vi "Control Panel.vi"(8 "error in (no error)":errorcluster, 11 "Fake Pulse Generator in":refnum<class "Pulse Generator.lvclass">) -> (0 "error out":errorcluster, 3 "Fake Pulse Generator out":refnum<class "Pulse Generator.lvclass">)   [LabVIEW 2009, in "Pulse Generator.lvclass"]
uses:
  Pulse Generator.lvclass
  Utility Classes/Scannable/Scannable.lvclass
  Pulse Generator.lvclass/Pulse Generator.ctl
panel:
  in  "Width/Duty\nUP/DOWN Ch2":bool
  in  "Width/Duty\nUP/DOWN Ch1":bool
  in  "Clear Error":bool
  out "Ready when \nblinking":bool
  in  "Copy actual to set":bool
  out "Pulse Mode":enum16{"Pulses", "Pattern"}(ring)
  out "Arming (Trigger) Source":T1(ring)
  in  "Populate fields with member data":bool
  out "Strobe Pattern":string
  in  "Strobe Pattern Set":string
  out "StrobeDataBuffer":digitalwaveform(graph)
  in  "Enable/disable":bool
  in  "Modes (changes immediately)":T2(radio)
  in  "BitPeriodSet":dbl[unit]
  out "BitPeriod":dbl[unit]
  out "Ch2Pattern":string
  in  "Ch2Pattern Set":string
  out "Ch1Pattern":string
  in  "Set Patterns":bool
  in  "Ch1Pattern Set":string
  in  "Ch2Duty (%) Set":dbl=10.0
  in  "Ch1Duty (%) Set":dbl=10.0
  in  "Ch1Delay Set":dbl[unit]
  in  "Ch2Delay Set":dbl[unit]
  in  "stop":bool
  out "Ch1DataBuffer":digitalwaveform(graph)
  out "Ch2DataBuffer":digitalwaveform(graph)
  in  "Ch2 Sync":bool
  in  "Ch1 Sync":bool
  in  "Ch2 Toggle":bool
  in  "Ch1 NOT Toggle":bool
  in  "Ch1 Toggle":bool
  in  "Ch2 NOT Toggle":bool
  in  "OverallPeriodSet":dbl[unit]
  in  "Ch2WidthSet":dbl[unit]=1e-09
  in  "Ch1WidthSet":dbl[unit]=1e-09
  in  "Ch2LowSet":dbl[unit]
  in  "Ch2HighSet":dbl[unit]
  in  "Ch1LowSet":dbl[unit]
  in  "Ch1HighSet":dbl[unit]
  in  "OverallFreqSet":dbl[unit]
  in  "Read to Control":bool
  in  "Set":bool
  out "Ch2Duty (%)":dbl
  out "Ch1Duty (%)":dbl
  out "Ch1Delay":dbl[unit]
  out "Ch2Delay":dbl[unit]
  out "Ch1Low":dbl[unit]
  out "Ch1High":dbl[unit]
  out "Ch2Width":dbl[unit]
  out "Ch1Width":dbl[unit]
  out "OverallPeriod":dbl[unit]
  out "Ch2Low":dbl[unit]
  out "Ch2High":dbl[unit]
  in  "Read":bool
  out "OverallFreq":dbl[unit]
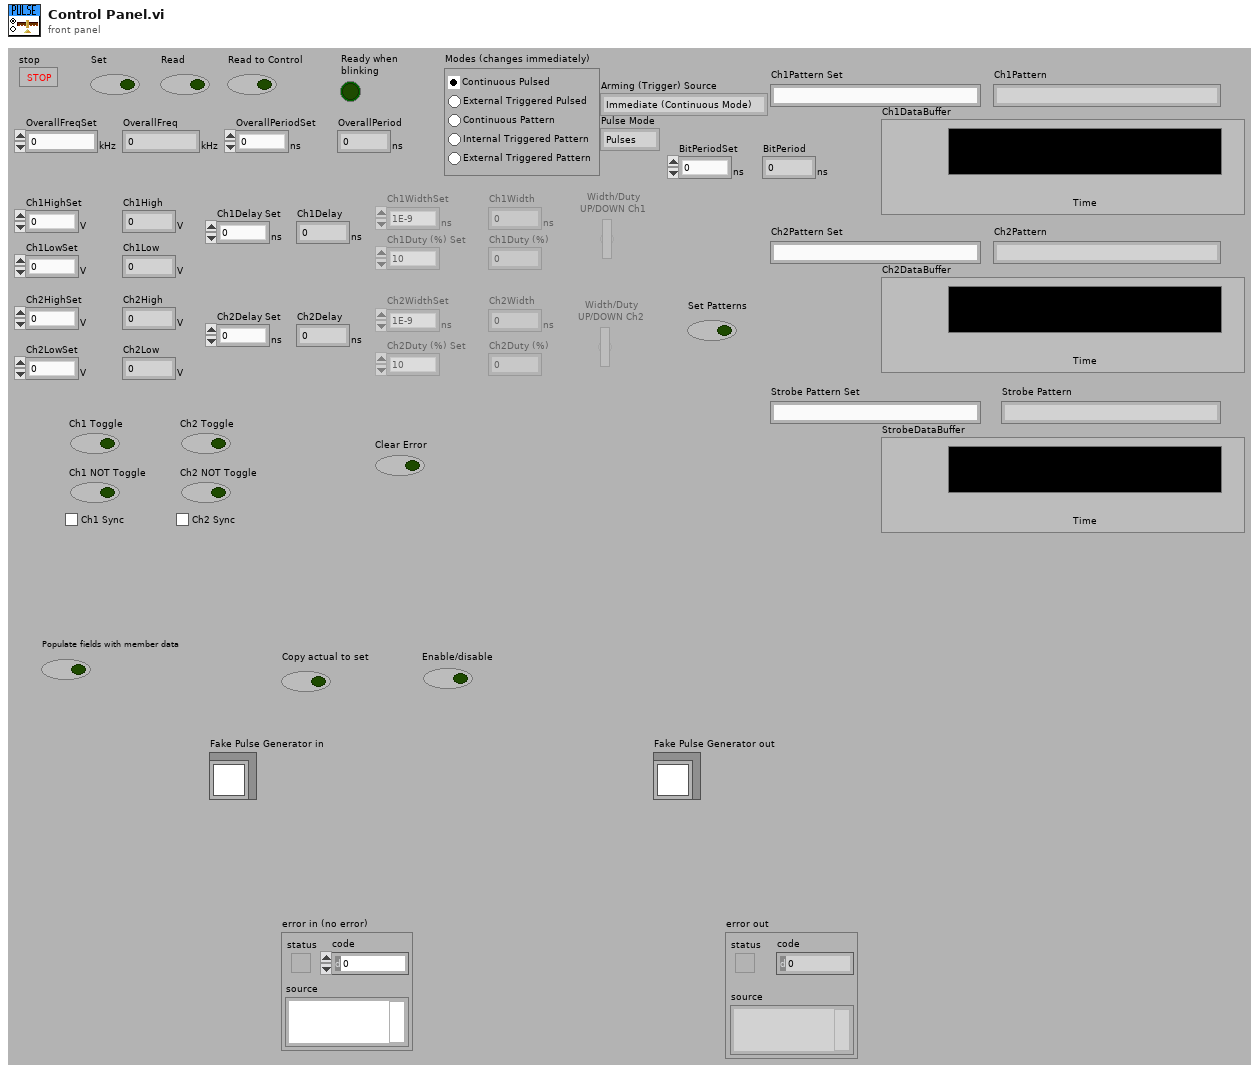
[diagram p1: front panel]
types:
  T1 = enum16{"Immediate (Continuous Mode)", "Internal PLL", "External", "Manual"}
  T2 = enum32{"Continuous Pulsed", "Continuous Pattern", "Internal Triggered Pattern", "External Triggered Pulsed", "External Triggered Pattern", "Other"}
  T3 = enum16{"Internal Oscillator", "Internal PLL", "External Clock "}
  T4 = enum16{"Internal Oscillator", "Internal PLL", "Clock Input"}
  T5 = enum16{"Channel All ", "Channel 1", "Channel 2", "Channel 3", "Channels Combined"}
  T6 = cluster{"1 High":dbl[unit], "1 Low":dbl[unit], "2 High":dbl[unit], "2 Low":dbl[unit]}
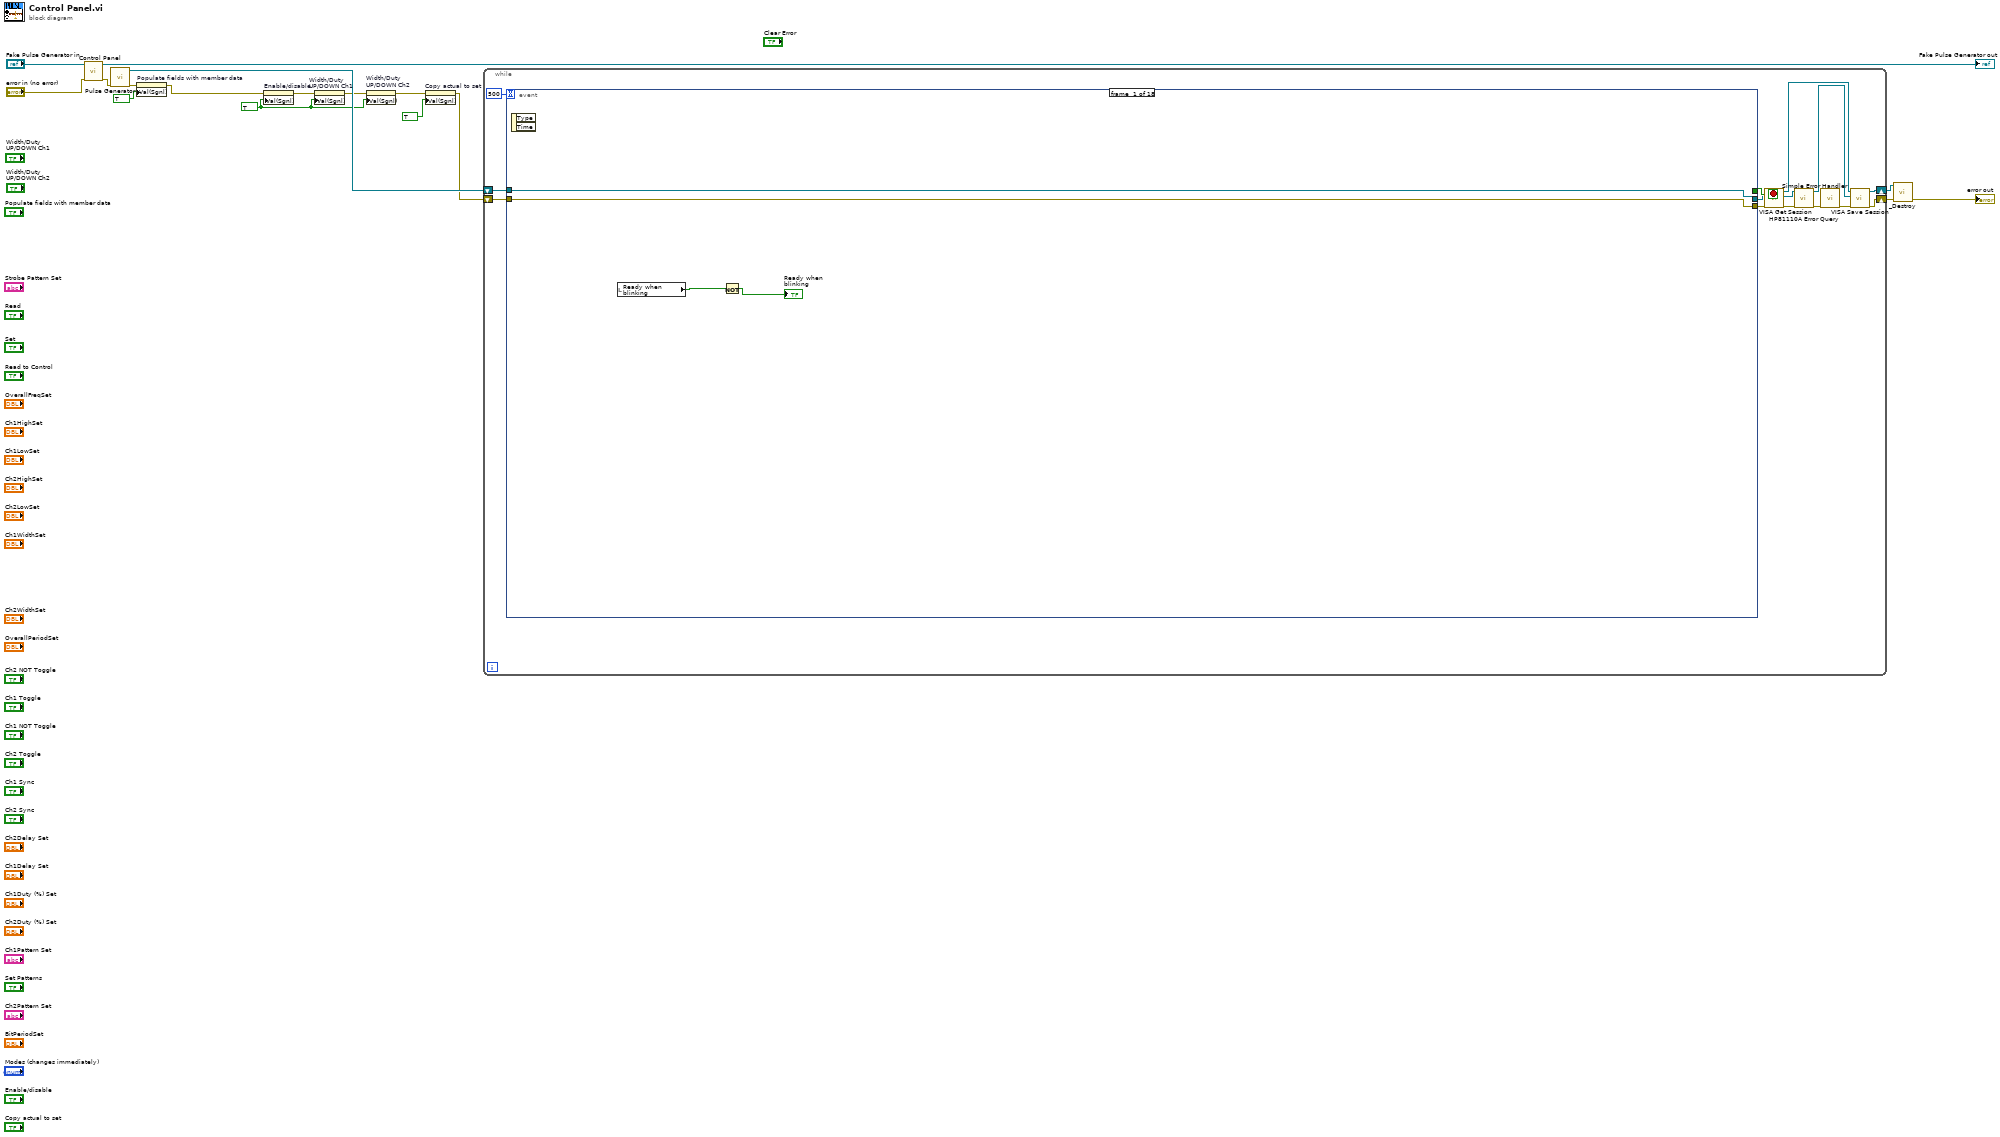
[diagram p0: block diagram]
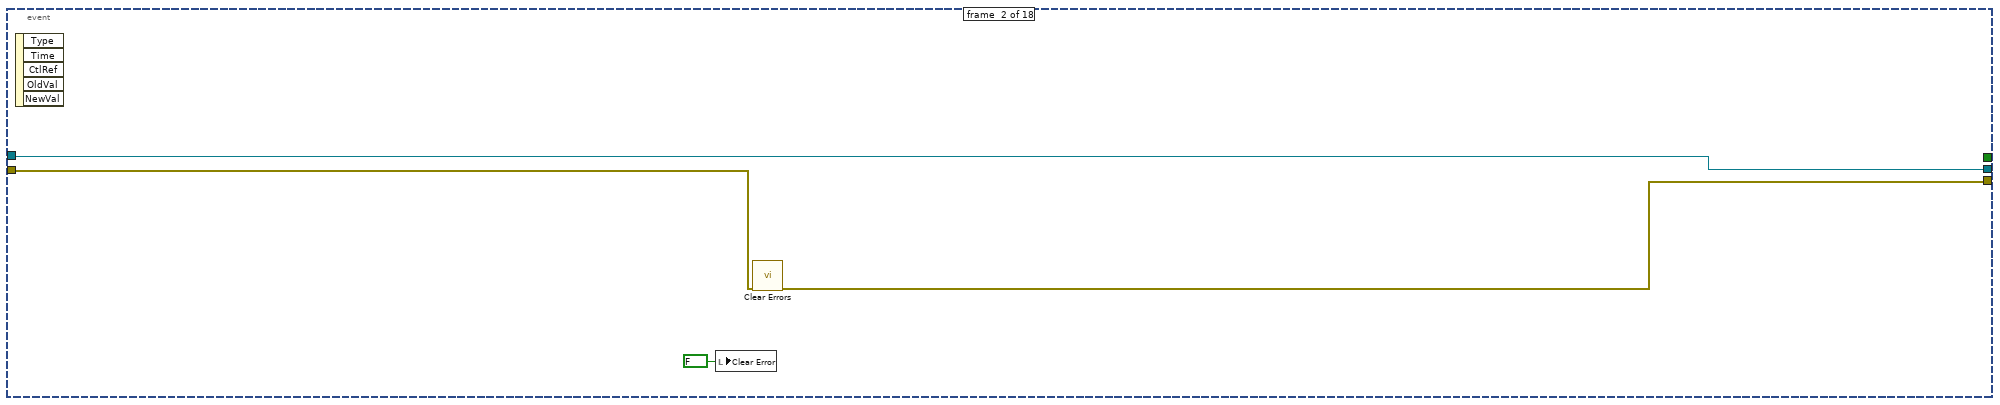
[diagram p2: hidden frame]
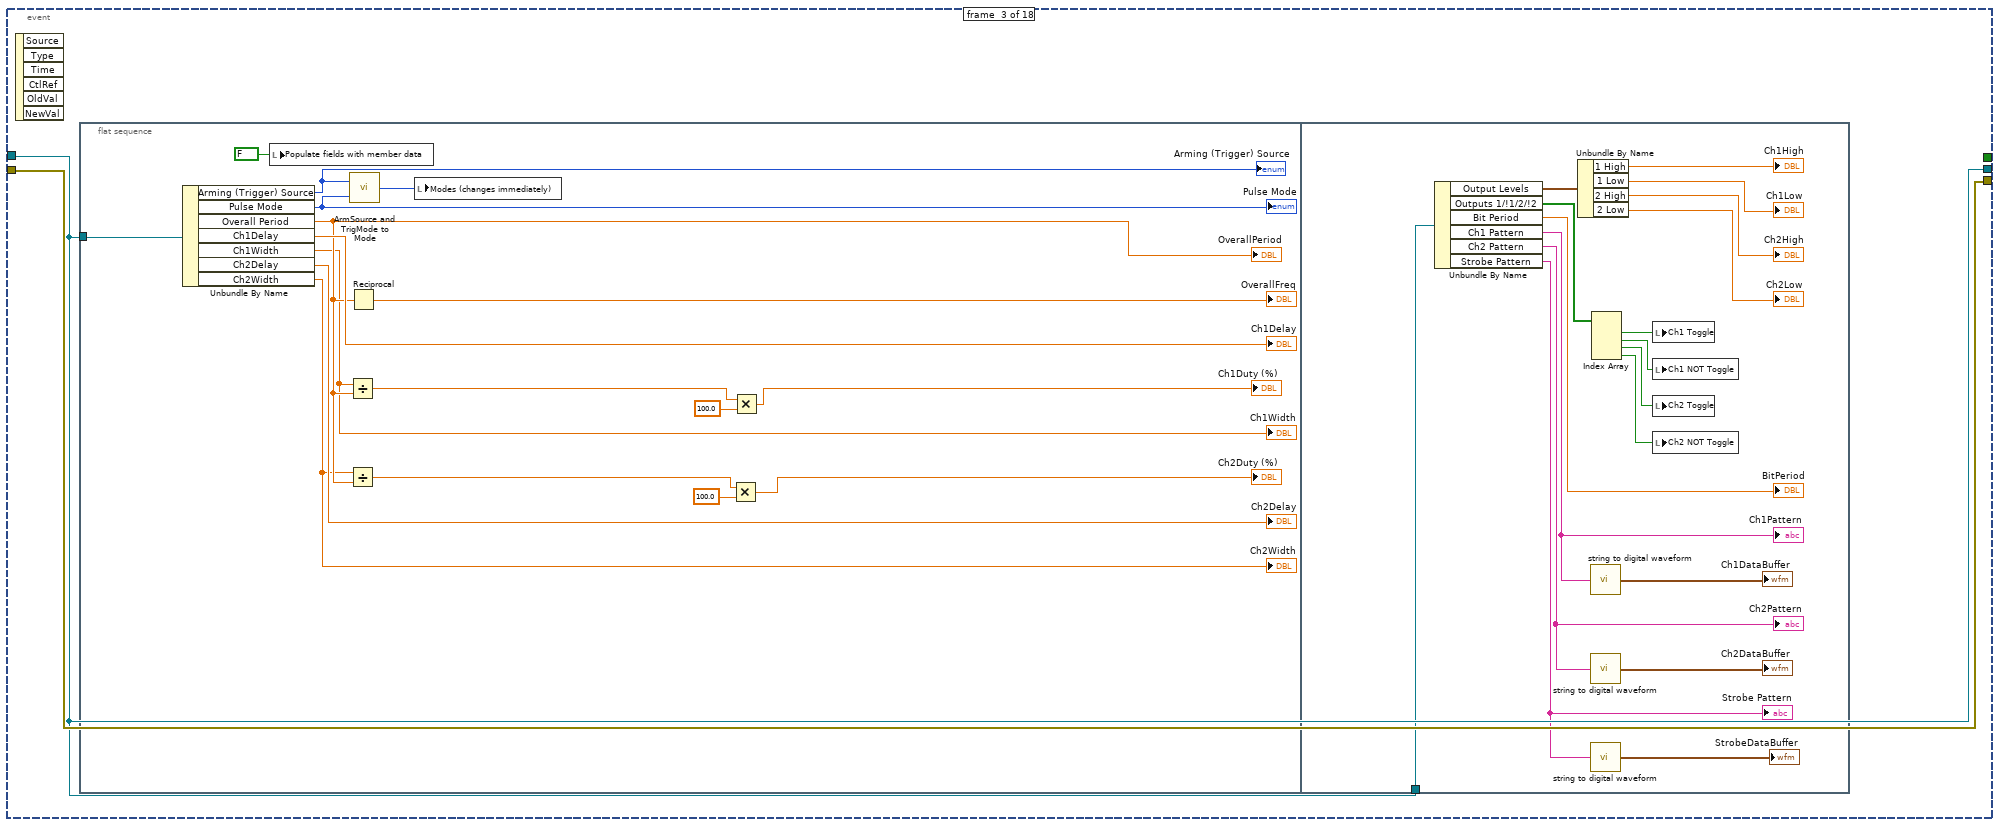
[diagram p3: hidden frame]
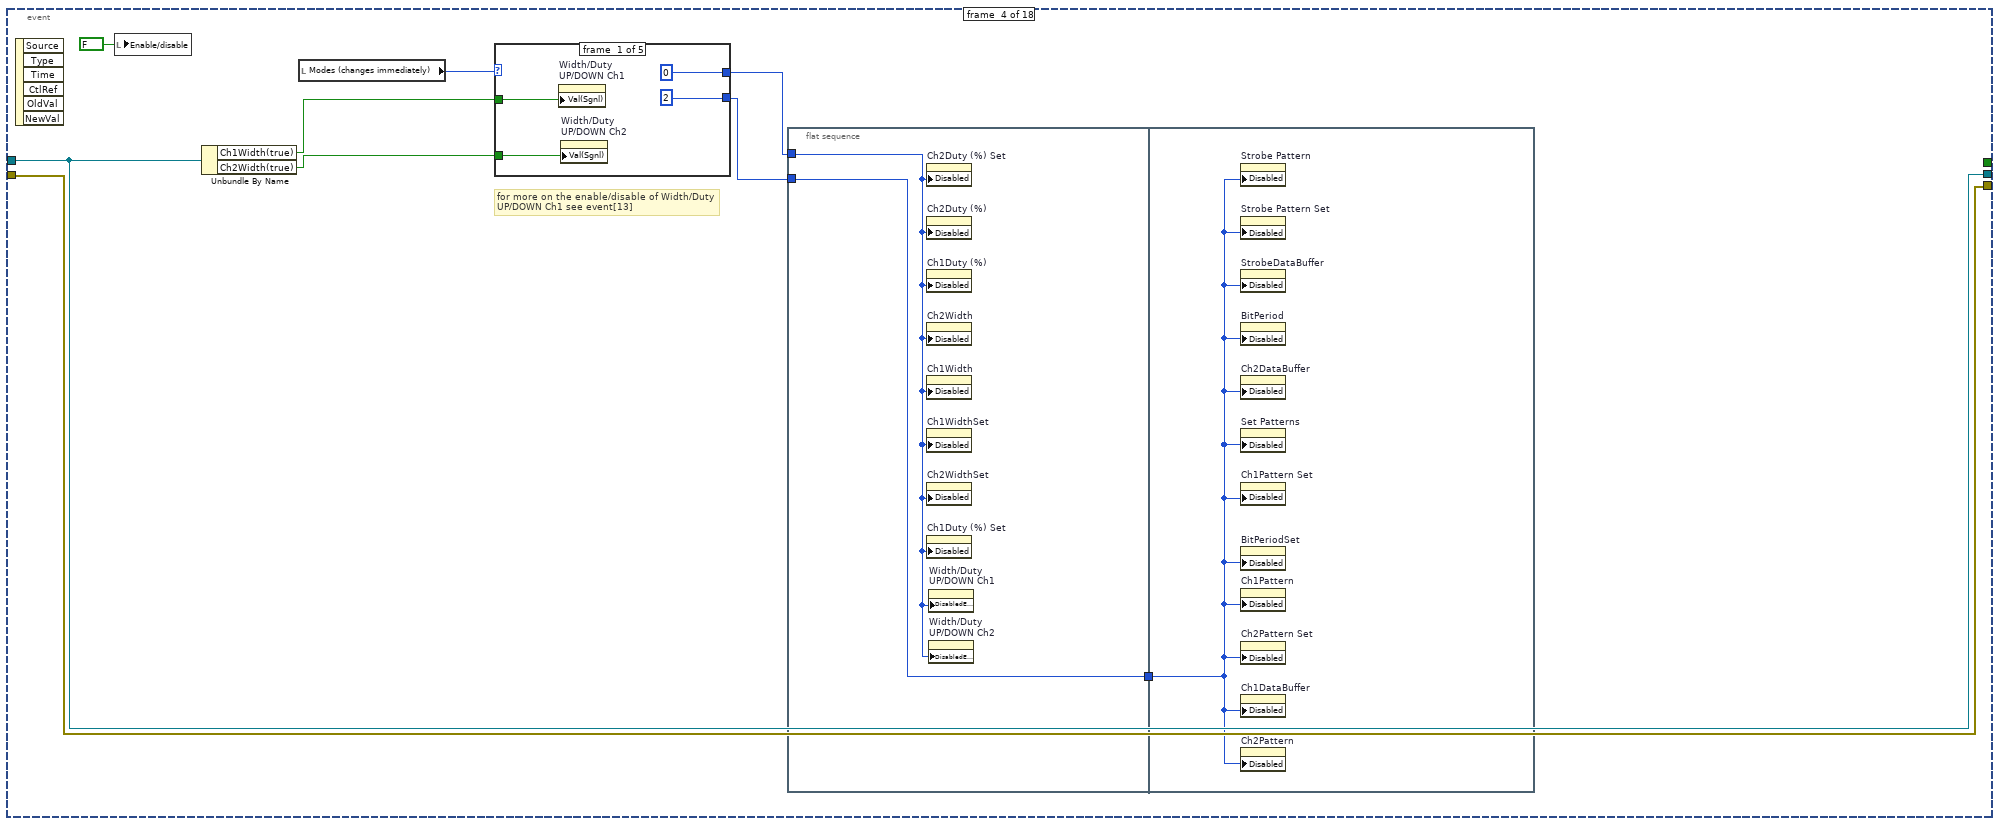
[diagram p4: hidden frame]
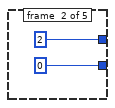
[diagram p5: hidden frame]
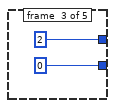
[diagram p6: hidden frame]
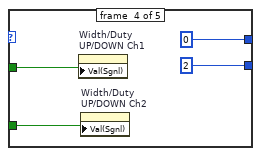
[diagram p7: hidden frame]
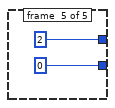
[diagram p8: hidden frame]
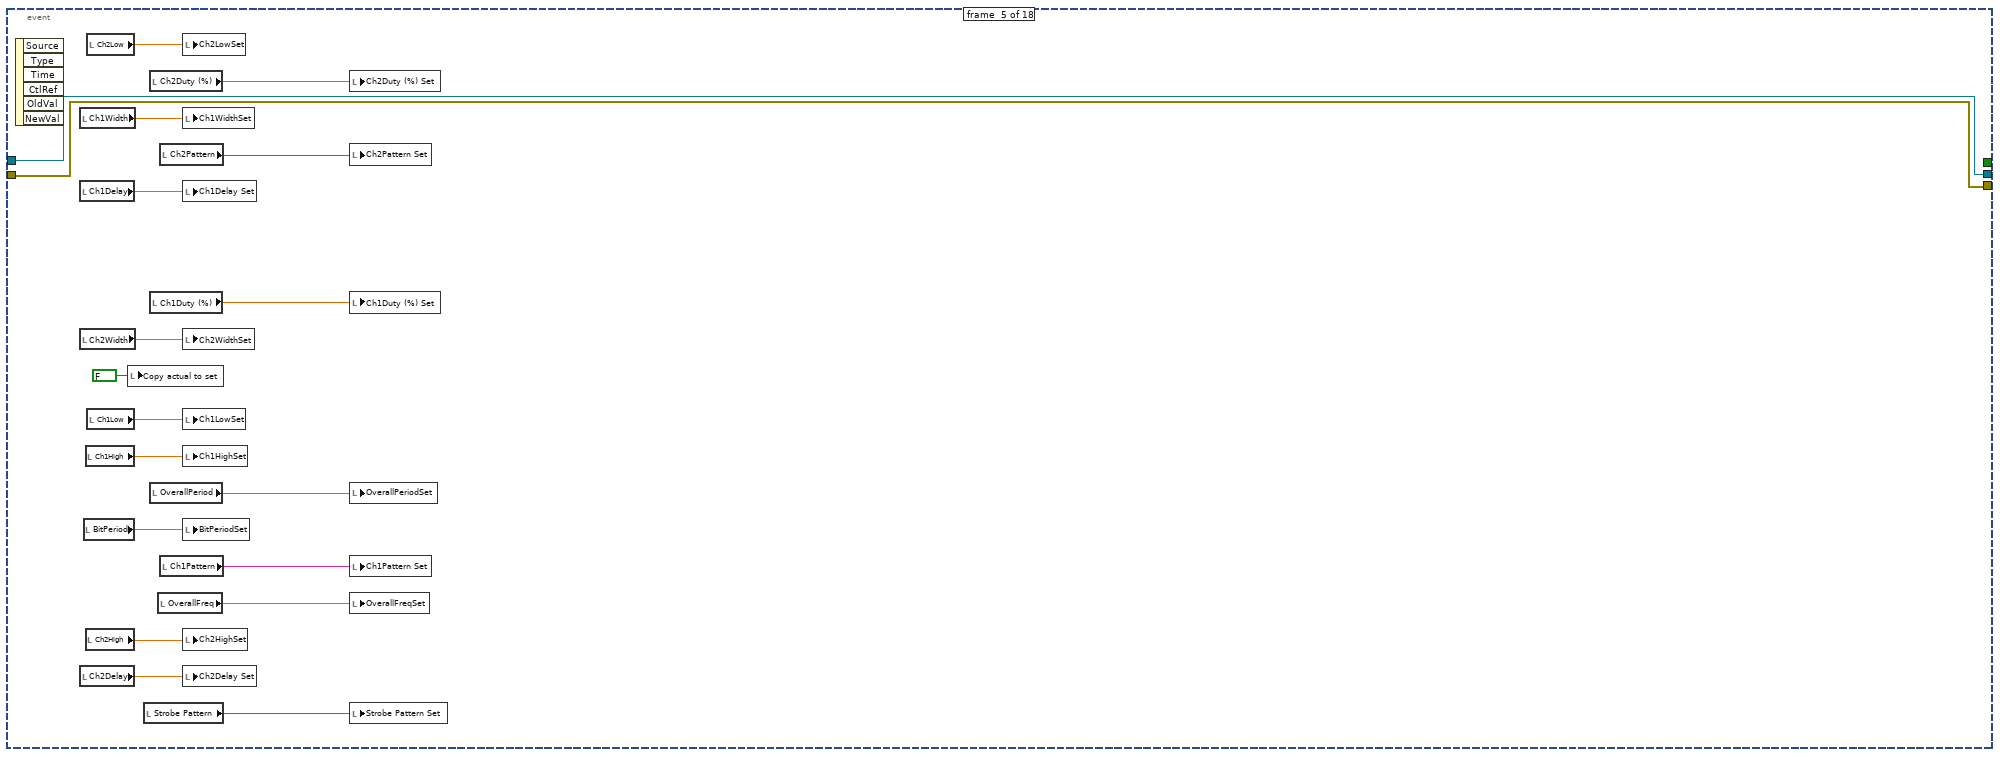
[diagram p9: hidden frame]
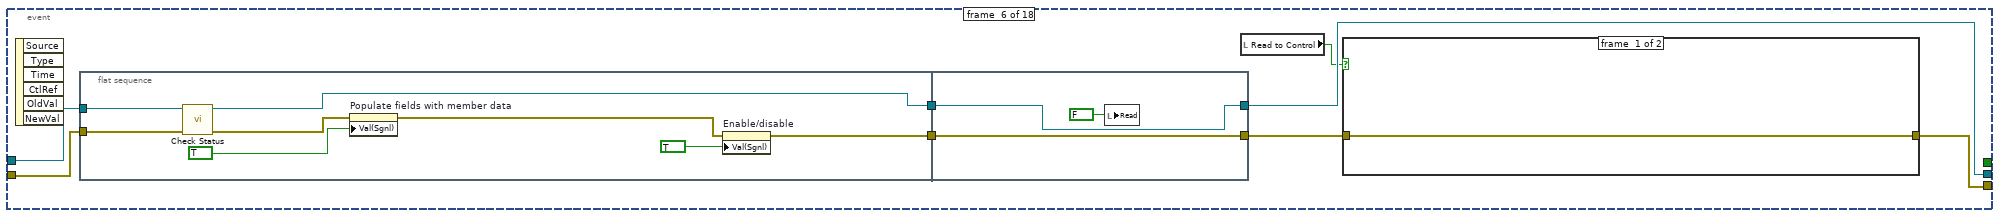
[diagram p10: hidden frame]
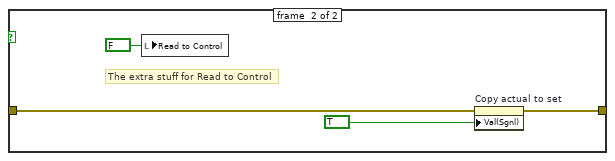
[diagram p11: hidden frame]
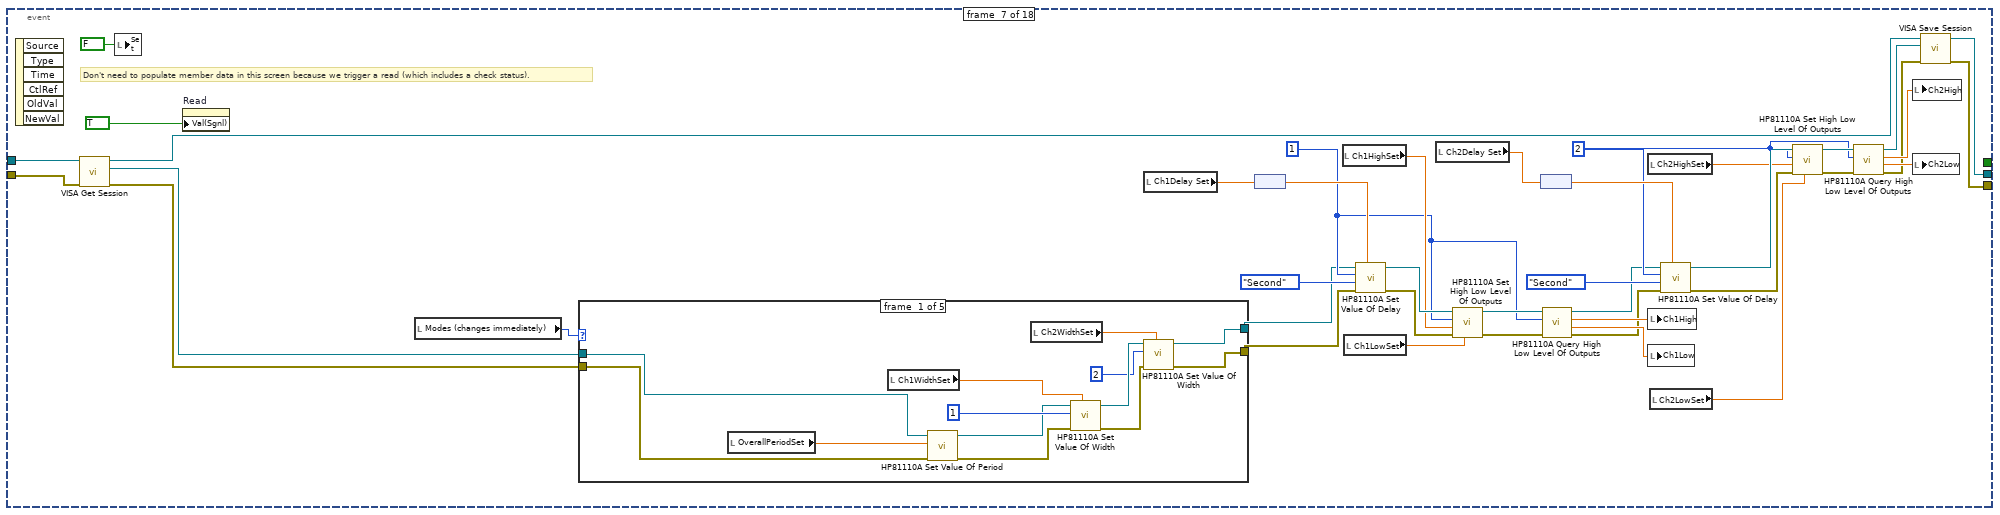
[diagram p12: hidden frame]
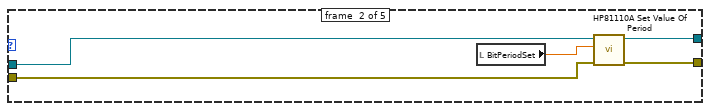
[diagram p13: hidden frame]
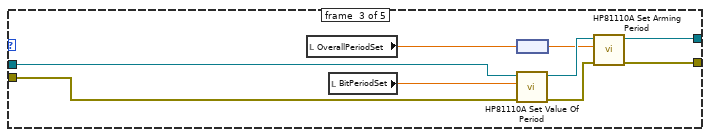
[diagram p14: hidden frame]
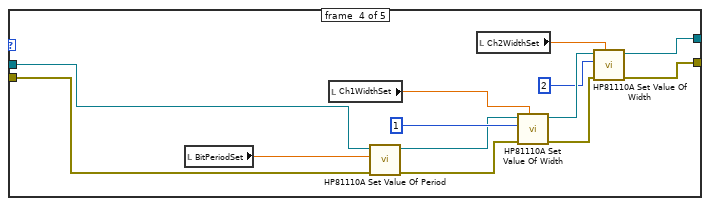
[diagram p15: hidden frame]
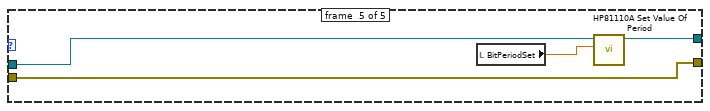
[diagram p16: hidden frame]
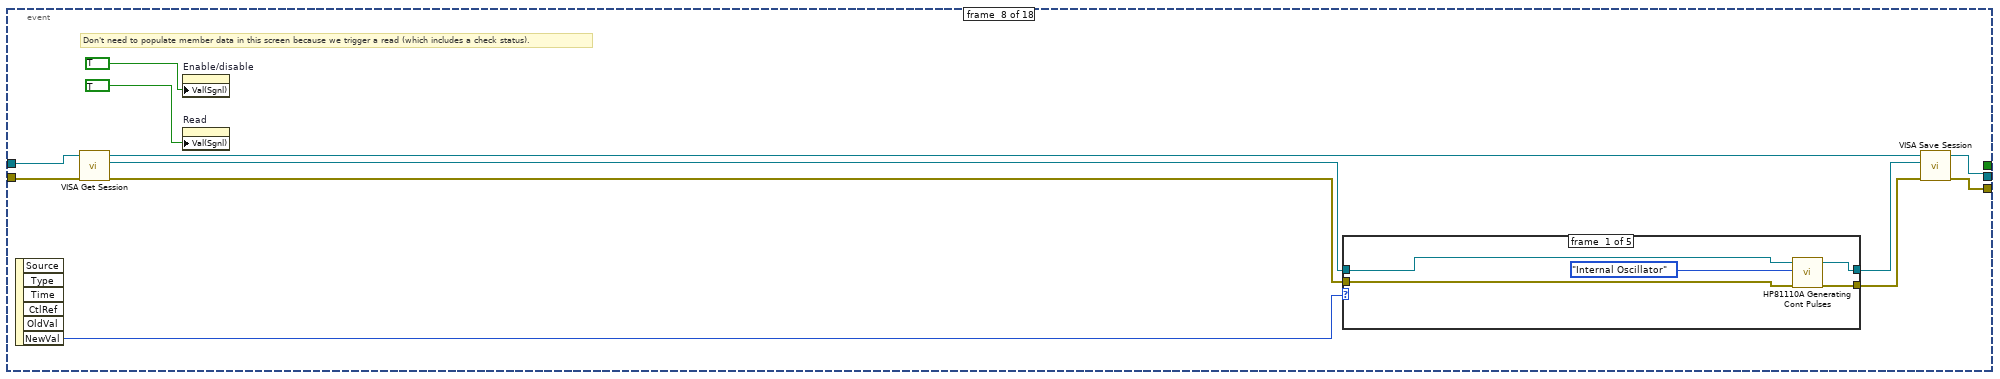
[diagram p17: hidden frame]
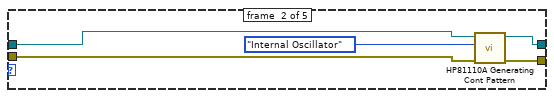
[diagram p18: hidden frame]
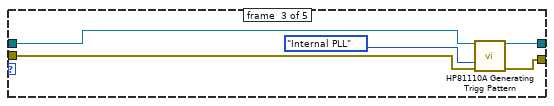
[diagram p19: hidden frame]
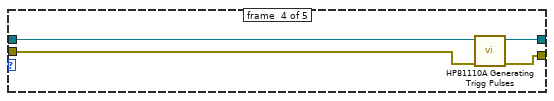
[diagram p20: hidden frame]
diagram:
  w1 = TRUE ("Value (Signaling)")
  n1 = call-parent "Control Panel.vi"("error in (no error)"="error in (no error)", "Instrument in"="Fake Pulse Generator in") -> ("error out"=w8:errorcluster, "Instrument out"=→"Fake Pulse Generator out":refnum<class "Pulse Generator.lvclass">)  [unwired: 8 out]
  n2 = call "Pulse Generator.vi"("error in (no error)"=w8) -> ("error out"=w9:errorcluster, "Pulse Generator out"=w14:refnum<class "Pulse Generator.lvclass">)  [unwired: 9 out]
  n3 = property on="Populate fields with member data" class="Bool (strict)"(error in=w9, "Val(Sgnl)"=TRUE ("Value (Signaling)")) -> (error out=w6:errorcluster)  [unwired: 1 in, 1 out]
  n4 = property on="Enable/disable" class="Bool (strict)"(error in=w6, "Val(Sgnl)"=w1) -> (error out=w4:errorcluster)  [unwired: 1 in, 1 out]
  n5 = property on="Width/Duty\nUP/DOWN Ch1" class="Bool (strict)"(error in=w4, "Val(Sgnl)"=w1) -> (error out=w2:errorcluster)  [unwired: 1 in, 1 out]
  n6 = property on="Width/Duty\nUP/DOWN Ch2" class="Bool (strict)"(error in=w2, "Val(Sgnl)"=w1) -> (error out=w3:errorcluster)  [unwired: 1 in, 1 out]
  n7 = property on="Copy actual to set" class="Bool (strict)"(error in=w3, "Val(Sgnl)"=TRUE ("Value (Signaling)")) -> (error out=w5:errorcluster)  [unwired: 1 in, 1 out]
  n8 = while {
    shift-right: [w24] -> w13
    shift-left: w14 -> [w29]
    shift-right: [w19] -> w12
    shift-left: w5 -> [w28]
    stop <- w31 stop-if-true
    n9 = event shown="[2] \"Populate fields with member data\": Value Change" {
      selector: _ -> [_ _ _ _ _ _ _ _ _ _ _ _ _ _ _ _ _ _]
      dyn-events: _ -> [_ _ _ _ _ _ _ _ _ _ _ _ _ _ _ _ _ _]
      timeout: 500 -> [_ _ _ _ _ _ _ _ _ _ _ _ _ _ _ _ _ _]
      tunnel: [_ _ _ _ _ _ _ _ _ _ _ _ "stop" _ _ _ _ _] -> w31
      tunnel: w28 -> [w34 w39 w41 w84 w104 w129 w152 w236 w274 w302 w312 w335 w348 w368 w370 w380 w390 w396]
      tunnel: [w34 w37 w41 w84 w104 w125 w147 w232 w268 w300 w312 w335 w348 w368 w370 w380 w390 w396] -> w22
      tunnel: w29 -> [w35 w38 w40 w79 w105 w128 w154 w238 w275 w303 w313 w336 w347 w355 w369 w379 w389 w397]
      tunnel: [w35 w38 w40 w79 w105 w127 w149 w233 w270 w291 w313 w336 w347 w354 w369 w379 w389 w397] -> w23
      event #0 {
        n10 = event-data() -> ()  [unwired: 3 out]
        n11 = local read "Ready when \nblinking"() -> (w33:bool)
        n12 = Not(x=w33) -> (.not. x?=→"Ready when \nblinking":bool)
      }
      event #1 {
        n13 = event-data() -> ()  [unwired: 6 out]
        n14 = local write "Clear Error"(FALSE ("Clear Error")) -> ()
        n15 = call <vilib>:"Clear Errors.vi"("error in (no error)"=w39) -> ("error out"=w37:errorcluster)  [unwired: 6 in]
      }
      event #2 {
        n16 = event-data() -> ()  [unwired: 7 out]
        n17 = flat-sequence {
          tunnel: w40 -> [w48]
          tunnel: w40 -> [w59]
          frame #0 {
            n18 = Unbundle By Name(w48) -> ("Arming (Trigger) Source"=w51:u16, "Pulse Mode"=w50:u16, "Overall Period"=w54:dbl[unit], "Ch1Delay"=→"Ch1Delay":dbl[unit], "Ch1Width"=w53:dbl[unit], "Ch2Delay"=→"Ch2Delay":dbl[unit], "Ch2Width"=w52:dbl[unit])
            "OverallPeriod" <- w54
            "Ch1Width" <- w53
            "Ch2Width" <- w52
            "Arming (Trigger) Source" <- w51
            "Pulse Mode" <- w50
            n19 = local write "Populate fields with member data"(FALSE ("Populate fields with member data")) -> ()
            n20 = Divide(x=w53, y=w54) -> (x/y=w45:dbl)
            n21 = Divide(x=w52, y=w54) -> (x/y=w43:dbl)
            n22 = Reciprocal(x=w54) -> (1/x=→"OverallFreq":dbl[unit])
            n23 = call "ArmSource and TrigMode to Mode.vi"("Pulse Mode"=w50, "Arming (Trigger) Source (0:Internal PLL)"=w51) -> ("Modes (changes immediately)"=w49:T2)
            n24 = local write "Modes (changes immediately)"(w49) -> ()
            n25 = Multiply(x=w43, y=100.0) -> (x*y=→"Ch2Duty (%)":dbl)
            n26 = Multiply(x=w45, y=100.0) -> (x*y=→"Ch1Duty (%)":dbl)
          }
          frame #1 {
            n27 = Unbundle By Name(w59) -> ("Output Levels"=w71:T6, "Outputs 1/!1/2/!2"=w72:bool[], "Bit Period"=→"BitPeriod":dbl[unit], "Ch1 Pattern"=w74:string, "Ch2 Pattern"=w75:string, "Strobe Pattern"=w76:string)
            "Ch1Pattern" <- w74
            "Ch2Pattern" <- w75
            "Strobe Pattern" <- w76
            n28 = Unbundle By Name(w71) -> ("1 High"=→"Ch1High":dbl[unit], "1 Low"=→"Ch1Low":dbl[unit], "2 High"=→"Ch2High":dbl[unit], "2 Low"=→"Ch2Low":dbl[unit])
            n29 = call "string to digital waveform.vi"("String"=w74) -> ("digital waveform"=→"Ch1DataBuffer":digitalwaveform)
            n30 = call "string to digital waveform.vi"("String"=w75) -> ("digital waveform"=→"Ch2DataBuffer":digitalwaveform)
            n31 = call "string to digital waveform.vi"("String"=w76) -> ("digital waveform"=→"StrobeDataBuffer":digitalwaveform)
            n32 = Index Array(array=w72) -> (element #1=w67:bool, element #2=w68:bool, element #3=w69:bool, element #4=w70:bool)  [unwired: 4 in]
            n33 = local write "Ch1 Toggle"(w67) -> ()
            n34 = local write "Ch1 NOT Toggle"(w68) -> ()
            n35 = local write "Ch2 Toggle"(w69) -> ()
            n36 = local write "Ch2 NOT Toggle"(w70) -> ()
          }
        }
      }
      event #3 {
        # "for more on the enable/disable of Width/Duty\nUP/DOWN Ch1 see event[13]"
        n37 = event-data() -> ()  [unwired: 7 out]
        n38 = local write "Enable/disable"(FALSE ("Enable/disable")) -> ()
        n39 = Unbundle By Name(w79) -> ("Ch1Width(true)"=w77:bool, "Ch2Width(true)"=w78:bool)
        n40 = local read "Modes (changes immediately)"() -> (w82:T2)
        n41 = case shown="\"External Triggered Pulsed\"" w82 {
          tunnel: [2 0 0 2 0] -> w80
          tunnel: [0 2 2 0 2] -> w81
          tunnel: w78 -> [w87 _ _ w94 _]
          tunnel: w77 -> [w86 _ _ w95 _]
          frame #0 {
            n42 = property on="Width/Duty\nUP/DOWN Ch1" class="Bool (strict)"("Val(Sgnl)"=w86) -> ()  [unwired: 2 in, 2 out]
            n43 = property on="Width/Duty\nUP/DOWN Ch2" class="Bool (strict)"("Val(Sgnl)"=w87) -> ()  [unwired: 2 in, 2 out]
          }
          frame #1 {
          }
          frame #2 {
          }
          frame #3 {
            n44 = property on="Width/Duty\nUP/DOWN Ch1" class="Bool (strict)"("Val(Sgnl)"=w95) -> ()  [unwired: 2 in, 2 out]
            n45 = property on="Width/Duty\nUP/DOWN Ch2" class="Bool (strict)"("Val(Sgnl)"=w94) -> ()  [unwired: 2 in, 2 out]
          }
          frame #4 {
          }
        }
        n46 = flat-sequence {
          tunnel: [w101] -> w83
          tunnel: w81 -> [w100]
          tunnel: w80 -> [w101]
          tunnel: w83 -> [w102]
          frame #0 {
            n47 = property on="Ch2Duty (%) Set" class="DigNum (strict)"("Disabled"=w100) -> ()  [unwired: 2 in, 2 out]
            n48 = property on="Ch2Duty (%)" class="DigNum (strict)"("Disabled"=w100) -> ()  [unwired: 2 in, 2 out]
            n49 = property on="Ch1Duty (%)" class="DigNum (strict)"("Disabled"=w100) -> ()  [unwired: 2 in, 2 out]
            n50 = property on="Ch2Width" class="DigNum (strict)"("Disabled"=w100) -> ()  [unwired: 2 in, 2 out]
            n51 = property on="Ch1Width" class="DigNum (strict)"("Disabled"=w100) -> ()  [unwired: 2 in, 2 out]
            n52 = property on="Ch1WidthSet" class="DigNum (strict)"("Disabled"=w100) -> ()  [unwired: 2 in, 2 out]
            n53 = property on="Ch2WidthSet" class="DigNum (strict)"("Disabled"=w100) -> ()  [unwired: 2 in, 2 out]
            n54 = property on="Ch1Duty (%) Set" class="DigNum (strict)"("Disabled"=w100) -> ()  [unwired: 2 in, 2 out]
            n55 = property on="Width/Duty\nUP/DOWN Ch1" class="Bool (strict)"("DisabledEnum"=w100) -> ()  [unwired: 2 in, 2 out]
            n56 = property on="Width/Duty\nUP/DOWN Ch2" class="Bool (strict)"("DisabledEnum"=w100) -> ()  [unwired: 2 in, 2 out]
          }
          frame #1 {
            n57 = property on="Strobe Pattern" class="Str"("Disabled"=w102) -> ()  [unwired: 2 in, 2 out]
            n58 = property on="Strobe Pattern Set" class="Str"("Disabled"=w102) -> ()  [unwired: 2 in, 2 out]
            n59 = property on="StrobeDataBuffer" class="DigitalGraph (strict)"("Disabled"=w102) -> ()  [unwired: 2 in, 2 out]
            n60 = property on="BitPeriod" class="DigNum (strict)"("Disabled"=w102) -> ()  [unwired: 2 in, 2 out]
            n61 = property on="Ch2DataBuffer" class="DigitalGraph (strict)"("Disabled"=w102) -> ()  [unwired: 2 in, 2 out]
            n62 = property on="Set Patterns" class="Bool (strict)"("Disabled"=w102) -> ()  [unwired: 2 in, 2 out]
            n63 = property on="Ch1Pattern Set" class="Str"("Disabled"=w102) -> ()  [unwired: 2 in, 2 out]
            n64 = property on="BitPeriodSet" class="DigNum (strict)"("Disabled"=w102) -> ()  [unwired: 2 in, 2 out]
            n65 = property on="Ch1Pattern" class="Str"("Disabled"=w102) -> ()  [unwired: 2 in, 2 out]
            n66 = property on="Ch2Pattern Set" class="Str"("Disabled"=w102) -> ()  [unwired: 2 in, 2 out]
            n67 = property on="Ch1DataBuffer" class="DigitalGraph (strict)"("Disabled"=w102) -> ()  [unwired: 2 in, 2 out]
            n68 = property on="Ch2Pattern" class="Str"("Disabled"=w102) -> ()  [unwired: 2 in, 2 out]
          }
        }
      }
      event #4 {
        n69 = event-data() -> ()  [unwired: 7 out]
        n70 = local read "Ch1Width"() -> (w117:dbl[unit])
        n71 = local read "Ch1Delay"() -> (w115:dbl[unit])
        n72 = local read "Ch2Width"() -> (w113:dbl[unit])
        n73 = local read "Ch2Delay"() -> (w111:dbl[unit])
        n74 = local read "BitPeriod"() -> (w107:dbl[unit])
        n75 = local read "Ch1High"() -> (w119:dbl[unit])
        n76 = local read "Ch2High"() -> (w110:dbl[unit])
        n77 = local read "Ch2Low"() -> (w114:dbl[unit])
        n78 = local read "Ch1Low"() -> (w118:dbl[unit])
        n79 = local write "Copy actual to set"(FALSE ("Copy actual to set")) -> ()
        n80 = local read "Strobe Pattern"() -> (w103:string)
        n81 = local read "Ch2Duty (%)"() -> (w112:dbl)
        n82 = local read "Ch1Duty (%)"() -> (w116:dbl)
        n83 = local read "OverallPeriod"() -> (w120:dbl[unit])
        n84 = local read "OverallFreq"() -> (w121:dbl[unit])
        n85 = local read "Ch2Pattern"() -> (w108:string)
        n86 = local read "Ch1Pattern"() -> (w109:string)
        n87 = local write "Ch2LowSet"(w114) -> ()
        n88 = local write "Ch1WidthSet"(w117) -> ()
        n89 = local write "Ch1Delay Set"(w115) -> ()
        n90 = local write "Ch2WidthSet"(w113) -> ()
        n91 = local write "Ch1LowSet"(w118) -> ()
        n92 = local write "Ch1HighSet"(w119) -> ()
        n93 = local write "BitPeriodSet"(w107) -> ()
        n94 = local write "Ch2HighSet"(w110) -> ()
        n95 = local write "Ch2Delay Set"(w111) -> ()
        n96 = local write "Ch2Duty (%) Set"(w112) -> ()
        n97 = local write "Ch2Pattern Set"(w108) -> ()
        n98 = local write "Ch1Duty (%) Set"(w116) -> ()
        n99 = local write "OverallPeriodSet"(w120) -> ()
        n100 = local write "Ch1Pattern Set"(w109) -> ()
        n101 = local write "OverallFreqSet"(w121) -> ()
        n102 = local write "Strobe Pattern Set"(w103) -> ()
      }
      event #5 {
        n103 = event-data() -> ()  [unwired: 7 out]
        n104 = flat-sequence {
          tunnel: w129 -> [w137]
          tunnel: w128 -> [w136]
          tunnel: [w135] -> w123
          tunnel: [w134] -> w122
          tunnel: [w139] -> w126
          tunnel: [w140] -> w127
          tunnel: w123 -> [w140]
          tunnel: w122 -> [w139]
          frame #0 {
            n105 = call-dynamic "Check Status.vi"("error in (no error)"=w137, "Pulse Generator in"=w136) -> ("error out"=w131:errorcluster, "Pulse Generator out"=w135:refnum<class "Pulse Generator.lvclass">)  [unwired: 8 out]
            n106 = property on="Populate fields with member data" class="Bool (strict)"(error in=w131, "Val(Sgnl)"=TRUE ("Value (Signaling)")) -> (error out=w130:errorcluster)  [unwired: 1 in, 1 out]
            n107 = property on="Enable/disable" class="Bool (strict)"(error in=w130, "Val(Sgnl)"=TRUE ("Value (Signaling)")) -> (error out=w134:errorcluster)  [unwired: 1 in, 1 out]
          }
          frame #1 {
            n108 = local write "Read"(FALSE) -> ()
          }
        }
        n109 = local read "Read to Control"() -> (w124:bool)
        n110 = case shown="True" w124 {
          tunnel: w126 -> [w141 w143]
          tunnel: [w141 w142] -> w125
          frame #0 {
          }
          frame #1 {
            # "The extra stuff for Read to Control"
            n111 = local write "Read to Control"(FALSE) -> ()
            n112 = property on="Copy actual to set" class="Bool (strict)"(error in=w143, "Val(Sgnl)"=TRUE ("Value (Signaling)")) -> (error out=w142:errorcluster)  [unwired: 1 in, 1 out]
          }
        }
      }
      event #6 {
        w160 = 1
        w165 = 2
        # "Don't need to populate member data in this screen because we trigger a read (which includes a check status)."
        n113 = event-data() -> ()  [unwired: 7 out]
        n114 = call-dynamic "VISA Get Session.vi"("error in (no error)"=w152, "Instrument.lvclass in"=w154) -> ("error out"=w151:errorcluster, "VISA Resource Name"=w153:refnum<visa-resource-name>, "Instrument.lvclass out"=w150:refnum<class "Pulse Generator.lvclass">)  [unwired: 7 out]
        n115 = local write "Set"(FALSE) -> ()
        n116 = property on="Read" class="Bool (strict)"("Val(Sgnl)"=TRUE ("Value (Signaling)")) -> ()  [unwired: 2 in, 2 out]
        n117 = local read "Modes (changes immediately)"() -> (w157:T2)
        n118 = case shown="\"Continuous Pulsed\", Default" w157 {
          tunnel: w153 -> [w191 w202 w207 w218 w228]
          tunnel: w151 -> [w190 w200 w205 w215 w226]
          tunnel: [w187 w201 w206 w216 w227] -> w156
          tunnel: [w186 w199 w204 w213 w226] -> w155
          frame #0 {
            n119 = local read "OverallPeriodSet"() -> (w198:dbl[unit])
            n120 = local read "Ch1WidthSet"() -> (w192:dbl[unit])
            n121 = call "HP81110A Set Value Of Period.vi"("error in (no error)"=w190, "Period Value"=w198, "VISA session"=w191) -> ("error out"=w188:errorcluster, "dup VISA session"=w189:refnum<visa-resource-name>)  [unwired: 7 out]
            n122 = local read "Ch2WidthSet"() -> (w194:dbl[unit])
            n123 = call "HP81110A Set Value Of Width.vi"("Width Value (100.0E-9)"=w192, "error in (no error)"=w188, "Channel (1:Channel 1)"=1, "VISA session"=w189) -> ("error out"=w197:errorcluster, "dup VISA session"=w196:refnum<visa-resource-name>)  [unwired: 1 in, 5 out]
            n124 = call "HP81110A Set Value Of Width.vi"("Width Value (100.0E-9)"=w194, "error in (no error)"=w197, "Channel (1:Channel 1)"=2, "VISA session"=w196) -> ("error out"=w186:errorcluster, "dup VISA session"=w187:refnum<visa-resource-name>)  [unwired: 1 in, 5 out]
          }
          frame #1 {
            n125 = local read "BitPeriodSet"() -> (w203:dbl[unit])
            n126 = call "HP81110A Set Value Of Period.vi"("error in (no error)"=w200, "Period Value"=w203, "VISA session"=w202) -> ("error out"=w199:errorcluster, "dup VISA session"=w201:refnum<visa-resource-name>)  [unwired: 7 out]
          }
          frame #2 {
            n127 = local read "OverallPeriodSet"() -> (w209:dbl[unit])
            n128 = local read "BitPeriodSet"() -> (w208:dbl[unit])
            n129 = node(w209) -> (w210:dbl)
            n130 = call "HP81110A Set Value Of Period.vi"("error in (no error)"=w205, "Period Value"=w208, "VISA session"=w207) -> ("error out"=w212:errorcluster, "dup VISA session"=w211:refnum<visa-resource-name>)  [unwired: 7 out]
            n131 = call "HP81110A Set Arming Period.vi"("error in (no error)"=w212, "Period Value (10.0E-6 Sec)"=w210, "VISA session"=w211) -> ("error out"=w204:errorcluster, "dup VISA session"=w206:refnum<visa-resource-name>)  [unwired: 7 out]
          }
          frame #3 {
            n132 = local read "BitPeriodSet"() -> (w219:dbl[unit])
            n133 = local read "Ch1WidthSet"() -> (w220:dbl[unit])
            n134 = call "HP81110A Set Value Of Period.vi"("error in (no error)"=w215, "Period Value"=w219, "VISA session"=w218) -> ("error out"=w214:errorcluster, "dup VISA session"=w217:refnum<visa-resource-name>)  [unwired: 7 out]
            n135 = local read "Ch2WidthSet"() -> (w222:dbl[unit])
            n136 = call "HP81110A Set Value Of Width.vi"("Width Value (100.0E-9)"=w220, "error in (no error)"=w214, "Channel (1:Channel 1)"=1, "VISA session"=w217) -> ("error out"=w225:errorcluster, "dup VISA session"=w224:refnum<visa-resource-name>)  [unwired: 1 in, 5 out]
            n137 = call "HP81110A Set Value Of Width.vi"("Width Value (100.0E-9)"=w222, "error in (no error)"=w225, "Channel (1:Channel 1)"=2, "VISA session"=w224) -> ("error out"=w213:errorcluster, "dup VISA session"=w216:refnum<visa-resource-name>)  [unwired: 1 in, 5 out]
          }
          frame #4 {
            n138 = local read "BitPeriodSet"() -> (w229:dbl[unit])
            n139 = call "HP81110A Set Value Of Period.vi"("Period Value"=w229, "VISA session"=w228) -> ("dup VISA session"=w227:refnum<visa-resource-name>)  [unwired: 1 in, 8 out]
          }
        }
        n140 = local read "Ch1Delay Set"() -> (w183:dbl[unit])
        n141 = node(w183) -> (w182:dbl)
        n142 = local read "Ch1HighSet"() -> (w169:dbl[unit])
        n143 = local read "Ch1LowSet"() -> (w168:dbl[unit])
        n144 = call "HP81110A Set Value Of Delay.vi"("Delay Value (0.0)"=w182, "error in (no error)"=w155, "Delay Unit (0:Second)"=enum16{"Second", "Percent", "Degree", "Radians"}."Second", "Channel (1:Channel 1)"=w160, "VISA session"=w156) -> ("error out"=w173:errorcluster, "dup VISA session"=w172:refnum<visa-resource-name>)  [unwired: 5 out]
        n145 = local read "Ch2Delay Set"() -> (w181:dbl[unit])
        n146 = call "HP81110A Set High Low Level Of Outputs.vi"("Value Low (-0.5 V)"=w168, "error in (no error)"=w173, "Value High (0.5 V)"=w169, "Channel (1:Channel 1)"=w160, "VISA session"=w172) -> ("error out"=w170:errorcluster, "dup VISA session"=w171:refnum<visa-resource-name>)  [unwired: 5 out]
        n147 = node(w181) -> (w180:dbl)
        n148 = call "HP81110A Query High Low Level Of Outputs.vi"("error in (no error)"=w170, "Channel (1:Channel 1)"=w160, "VISA session"=w171) -> ("error out"=w158:errorcluster, "Value Low"=w166:dbl[unit], "Value High"=w167:dbl[unit], "dup VISA session"=w159:refnum<visa-resource-name>)  [unwired: 5 out]
        n149 = local read "Ch2HighSet"() -> (w164:dbl[unit])
        n150 = local write "Ch1High"(w167) -> ()
        n151 = local write "Ch1Low"(w166) -> ()
        n152 = local read "Ch2LowSet"() -> (w163:dbl[unit])
        n153 = call "HP81110A Set Value Of Delay.vi"("Delay Value (0.0)"=w180, "error in (no error)"=w158, "Delay Unit (0:Second)"=enum16{"Second", "Percent", "Degree", "Radians"}."Second", "Channel (1:Channel 1)"=w165, "VISA session"=w159) -> ("error out"=w175:errorcluster, "dup VISA session"=w177:refnum<visa-resource-name>)  [unwired: 5 out]
        n154 = call "HP81110A Set High Low Level Of Outputs.vi"("Value Low (-0.5 V)"=w163, "error in (no error)"=w175, "Value High (0.5 V)"=w164, "Channel (1:Channel 1)"=w165, "VISA session"=w177) -> ("error out"=w174:errorcluster, "dup VISA session"=w176:refnum<visa-resource-name>)  [unwired: 5 out]
        n155 = call "HP81110A Query High Low Level Of Outputs.vi"("error in (no error)"=w174, "Channel (1:Channel 1)"=w165, "VISA session"=w176) -> ("error out"=w148:errorcluster, "Value Low"=w161:dbl[unit], "Value High"=w162:dbl[unit], "dup VISA session"=w146:refnum<visa-resource-name>)  [unwired: 5 out]
        n156 = local write "Ch2High"(w162) -> ()
        n157 = local write "Ch2Low"(w161) -> ()
        n158 = call-dynamic "VISA Save Session.vi"("error in (no error)"=w148, "VISA Resource Name"=w146, "Instrument.lvclass in"=w150) -> ("error out"=w147:errorcluster, "Instrument.lvclass out"=w149:refnum<class "Pulse Generator.lvclass">)  [unwired: 7 out]
      }
      event #7 {
        # "Don't need to populate member data in this screen because we trigger a read (which includes a check status)."
        n159 = event-data() -> ("NewVal"=w241:T2)  [unwired: 6 out]
        n160 = call-dynamic "VISA Get Session.vi"("error in (no error)"=w236, "Instrument.lvclass in"=w238) -> ("error out"=w235:errorcluster, "VISA Resource Name"=w237:refnum<visa-resource-name>, "Instrument.lvclass out"=w234:refnum<class "Pulse Generator.lvclass">)  [unwired: 7 out]
        n161 = property on="Enable/disable" class="Bool (strict)"("Val(Sgnl)"=TRUE ("Value (Signaling)")) -> ()  [unwired: 2 in, 2 out]
        n162 = property on="Read" class="Bool (strict)"("Val(Sgnl)"=TRUE ("Value (Signaling)")) -> ()  [unwired: 2 in, 2 out]
        n163 = case shown="\"Continuous Pulsed\", Default" w241 {
          tunnel: w237 -> [w245 w251 w255 w260 w264]
          tunnel: w235 -> [w244 w250 w254 w259 w263]
          tunnel: [w243 w249 w253 w258 w262] -> w231
          tunnel: [w242 w247 w252 w257 w261] -> w230
          frame #0 {
            n164 = call "HP81110A Generating Cont Pulses.vi"("error in (no error)"=w244, "Period Source (0:Internal)"=T3."Internal Oscillator", "VISA session"=w245) -> ("error out"=w243:errorcluster, "dup VISA session"=w242:refnum<visa-resource-name>)  [unwired: 1 in, 6 out]
          }
          frame #1 {
            n165 = call "HP81110A Generating Cont Pattern.vi"("error in (no error)"=w250, "Period Source (0:Internal Oscillator)"=T4."Internal Oscillator", "VISA session"=w251) -> ("error out"=w249:errorcluster, "dup VISA session"=w247:refnum<visa-resource-name>)  [unwired: 1 in, 6 out]
          }
          frame #2 {
            n166 = call "HP81110A Generating Trigg Pattern.vi"("VISA session"=w255, "Trigger Source (0:Internal PLL)"=enum16{"Internal PLL", "External", "Manual"}."Internal PLL", "error in (no error)"=w254) -> ("dup VISA session"=w252:refnum<visa-resource-name>, "error out"=w253:errorcluster)  [unwired: 5 in, 6 out]
          }
          frame #3 {
            n167 = call "HP81110A Generating Trigg Pulses.vi"("error in (no error)"=w259, "VISA session"=w260) -> ("error out"=w258:errorcluster, "dup VISA session"=w257:refnum<visa-resource-name>)  [unwired: 2 in, 6 out]
          }
          frame #4 {
            n168 = call "HP81110A Generating Trigg Pattern.vi"("VISA session"=w264, "Period Source (0:Internal Oscillator)"=T4."Internal Oscillator", "Trigger Source (0:Internal PLL)"=enum16{"Internal PLL", "External", "Manual"}."External", "error in (no error)"=w263) -> ("dup VISA session"=w261:refnum<visa-resource-name>, "error out"=w262:errorcluster)  [unwired: 4 in, 6 out]
          }
        }
        n169 = call-dynamic "VISA Save Session.vi"("error in (no error)"=w231, "VISA Resource Name"=w230, "Instrument.lvclass in"=w234) -> ("error out"=w232:errorcluster, "Instrument.lvclass out"=w233:refnum<class "Pulse Generator.lvclass">)  [unwired: 7 out]
      }
      event #8 {
        # "Don't need to populate member data in this screen because we trigger a read (which includes a check status)."
        n170 = event-data() -> ()  [unwired: 7 out]
        n171 = local write "Set Patterns"(FALSE) -> ()
        n172 = property on="Read" class="Bool (strict)"("Val(Sgnl)"=TRUE ("Value (Signaling)")) -> ()  [unwired: 2 in, 2 out]
        n173 = local read "Strobe Pattern Set"() -> (w277:string)
        n174 = local read "Ch1Pattern Set"() -> (w279:string)
        n175 = local read "Ch2Pattern Set"() -> (w278:string)
        n176 = call "three string merge.vi"("Strobe String (def: 10)"=w277, "Ch2 String"=w278, "Ch1 String"=w279) -> ("Merged Output String"=w276:string)  [unwired: 8 out]
        n177 = call-dynamic "VISA Get Session.vi"("error in (no error)"=w274, "Instrument.lvclass in"=w275) -> ("error out"=w273:errorcluster, "VISA Resource Name"=w272:refnum<visa-resource-name>, "Instrument.lvclass out"=w271:refnum<class "Pulse Generator.lvclass">)  [unwired: 7 out]
        n178 = call "HP81110A Transfer String Into Memory.vi"("error in (no error)"=w273, "String"=w276, "Channel (1:Channel 1)"=T5."Channels Combined", "VISA session"=w272) -> ("error out"=w280:errorcluster, "dup VISA session"=w281:refnum<visa-resource-name>)  [unwired: 6 out]
        n179 = call "HP81110A Set Update Mode Of Pattern Data.vi"("error in (no error)"=w280, "Pattern Update Mode (1:Continuous)"=enum16{"Off", "Continuous", "Once"}."Once", "VISA session"=w281) -> ("error out"=w269:errorcluster, "dup VISA session"=w267:refnum<visa-resource-name>)  [unwired: 7 out]
        n180 = call-dynamic "VISA Save Session.vi"("error in (no error)"=w269, "VISA Resource Name"=w267, "Instrument.lvclass in"=w271) -> ("error out"=w268:errorcluster, "Instrument.lvclass out"=w270:refnum<class "Pulse Generator.lvclass">)  [unwired: 7 out]
      }
      event #9 {
        n181 = event-data() -> ()  [unwired: 7 out]
        n182 = local read "Ch1 NOT Toggle"() -> (w298:bool)
        n183 = local read "Ch2 NOT Toggle"() -> (w297:bool)
        n184 = local read "Ch2 Toggle"() -> (w287:bool)
        n185 = local read "Ch1 Toggle"() -> (w289:bool)
        n186 = local read "Ch1 Sync"() -> (w304:bool)
        n187 = local read "Ch2 Sync"() -> (w299:bool)
        n188 = case shown="True" w304 {
          tunnel: [w307 w308] -> w288
          tunnel: w298 -> [w307 _]
          tunnel: w289 -> [_ w308]
          frame #0 {
          }
          frame #1 {
            n189 = local write "Ch1 NOT Toggle"(w308) -> ()
          }
        }
        n190 = case shown="True" w299 {
          tunnel: [w305 w306] -> w286
          tunnel: w297 -> [w305 _]
          tunnel: w287 -> [_ w306]
          frame #0 {
          }
          frame #1 {
            n191 = local write "Ch2 NOT Toggle"(w306) -> ()
          }
        }
        n192 = call-dynamic "VISA Get Session.vi"("error in (no error)"=w302, "Instrument.lvclass in"=w303) -> ("error out"=w295:errorcluster, "VISA Resource Name"=w296:refnum<visa-resource-name>, "Instrument.lvclass out"=w301:refnum<class "Pulse Generator.lvclass">)  [unwired: 7 out]
        n193 = call "HP81110A Output Set - Fast.vi"("notoutput2"=w286, "output1"=w289, "error in (no error)"=w295, "output2"=w287, "notoutput1"=w288, "VISA session"=w296) -> ("error out"=w293:errorcluster, "dup VISA session"=w294:refnum<visa-resource-name>)  [unwired: 4 out]
        n194 = call-dynamic "VISA Save Session.vi"("error in (no error)"=w293, "VISA Resource Name"=w294, "Instrument.lvclass in"=w301) -> ("error out"=w300:errorcluster, "Instrument.lvclass out"=w292:refnum<class "Pulse Generator.lvclass">)  [unwired: 7 out]
        n195 = Build Array(w289, w288, w287, w286) -> (w290:bool[])
        n196 = Bundle By Name(cluster=w292, "Outputs 1/!1/2/!2"=w290) -> (w291:refnum<class "Pulse Generator.lvclass">)
      }
      event #10 {
        n197 = event-data() -> ("NewVal"=w309:dbl[unit])  [unwired: 6 out]
        n198 = Reciprocal(x=w309) -> (1/x=w314:dbl[unit])
        n199 = local write "OverallFreqSet"(w314) -> ()
        n200 = local read "Width/Duty\nUP/DOWN Ch2"() -> (w310:bool)
        n201 = local read "Width/Duty\nUP/DOWN Ch1"() -> (w311:bool)
        n202 = case shown="True" w311 {
          tunnel: w309 -> [w327 w330]
          frame #0 {
            n203 = local read "Ch1Duty (%) Set"() -> (w325:dbl)
            n204 = Divide(x=w325, y=100.0) -> (x/y=w328:dbl)
            n205 = Multiply(x=w328, y=w327) -> (x*y=w326:dbl[unit])
            n206 = local write "Ch1Width"(w326) -> ()
          }
          frame #1 {
            n207 = local read "Ch1Width"() -> (w331:dbl[unit])
            n208 = Divide(x=w331, y=w330) -> (x/y=w334:dbl)
            n209 = Multiply(x=w334, y=100) -> (x*y=w333:dbl)
            n210 = local write "Ch1Duty (%) Set"(w333) -> ()
          }
        }
        n211 = case shown="True" w310 {
          tunnel: w309 -> [w316 w324]
          frame #0 {
            n212 = local read "Ch2Duty (%) Set"() -> (w319:dbl)
            n213 = Divide(x=w319, y=100.0) -> (x/y=w318:dbl)
            n214 = Multiply(x=w318, y=w316) -> (x*y=w315:dbl[unit])
            n215 = local write "Ch2Width"(w315) -> ()
          }
          frame #1 {
            n216 = local read "Ch2Width"() -> (w323:dbl[unit])
            n217 = Divide(x=w323, y=w324) -> (x/y=w322:dbl)
            n218 = Multiply(x=w322, y=100) -> (x*y=w320:dbl)
            n219 = local write "Ch2Duty (%) Set"(w320) -> ()
          }
        }
      }
      event #11 {
        n220 = event-data() -> ("NewVal"=w346:dbl[unit])  [unwired: 6 out]
        n221 = local read "Ch1Width"() -> (w345:dbl[unit])
        n222 = local read "Ch2Width"() -> (w344:dbl[unit])
        n223 = Reciprocal(x=w346) -> (1/x=w343:dbl[unit])
        n224 = Divide(x=w345, y=w343) -> (x/y=w340:dbl)
        n225 = Divide(x=w344, y=w343) -> (x/y=w338:dbl)
        n226 = local write "OverallPeriodSet"(w343) -> ()
        n227 = Multiply(x=w340, y=100) -> (x*y=w339:dbl)
        n228 = Multiply(x=w338, y=100) -> (x*y=w337:dbl)
        n229 = local write "Ch1Duty (%) Set"(w339) -> ()
        n230 = local write "Ch2Duty (%) Set"(w337) -> ()
      }
      event #12 {
        n231 = event-data() -> ()  [unwired: 7 out]
      }
      event #13 {
        n232 = event-data() -> ()  [unwired: 7 out]
        n233 = local read "Width/Duty\nUP/DOWN Ch1"() -> (w359:bool)
        n234 = local read "Width/Duty\nUP/DOWN Ch2"() -> (w356:bool)
        n235 = local read "Width/Duty\nUP/DOWN Ch1"() -> (w357:bool)
        n236 = local read "Width/Duty\nUP/DOWN Ch2"() -> (w358:bool)
        n237 = Bundle By Name(cluster=w355, "Ch1Width(true)"=w357, "Ch2Width(true)"=w356) -> (w354:refnum<class "Pulse Generator.lvclass">)
        n238 = Select(t=2, s=w359, f=0) -> (s? t:f=w350:i32)
        n239 = Select(t=2, s=w358, f=0) -> (s? t:f=w351:i32)
        n240 = Select(t=0, s=w356, f=2) -> (s? t:f=w352:i32)
        n241 = Select(t=0, s=w357, f=2) -> (s? t:f=w353:i32)
        n242 = property on="Ch1Duty (%) Set" class="DigNum (strict)"("Disabled"=w350) -> ()  [unwired: 2 in, 2 out]
        n243 = property on="Ch2Duty (%) Set" class="DigNum (strict)"("Disabled"=w351) -> ()  [unwired: 2 in, 2 out]
        n244 = property on="Ch2WidthSet" class="DigNum (strict)"("DisabledEnum"=w352) -> ()  [unwired: 2 in, 2 out]
        n245 = property on="Ch1WidthSet" class="DigNum (strict)"("DisabledEnum"=w353) -> ()  [unwired: 2 in, 2 out]
        n246 = property on="Ch2Duty (%)" class="DigNum (strict)"("Disabled"=w351) -> ()  [unwired: 2 in, 2 out]
        n247 = property on="Ch2Width" class="DigNum (strict)"("DisabledEnum"=w352) -> ()  [unwired: 2 in, 2 out]
        n248 = property on="Ch1Width" class="DigNum (strict)"("DisabledEnum"=w353) -> ()  [unwired: 2 in, 2 out]
        n249 = property on="Ch1Duty (%)" class="DigNum (strict)"("Disabled"=w350) -> ()  [unwired: 2 in, 2 out]
      }
      event #14 {
        # "this hard codes to have the duty cycle be read as a width"
        n250 = event-data() -> ()  [unwired: 7 out]
        n251 = local read "Ch1WidthSet"() -> (w373:dbl[unit])
        n252 = local read "Ch1Duty (%) Set"() -> (w377:dbl)
        n253 = local read "OverallPeriodSet"() -> (w375:dbl[unit])
        n254 = local read "Width/Duty\nUP/DOWN Ch1"() -> (w372:bool)
        n255 = Divide(x=w377, y=100.0) -> (x/y=w376:dbl)
        n256 = Multiply(x=w376, y=w375) -> (x*y=w374:dbl[unit])
        n257 = Select(t=w373, s=w372, f=w374) -> (s? t:f=w371:dbl[unit])
        n258 = local write "Ch1WidthSet"(w371) -> ()
      }
      event #15 {
        # "this hard codes to have the duty cycle be read as a width"
        n259 = event-data() -> ()  [unwired: 7 out]
        n260 = local read "Ch2WidthSet"() -> (w382:dbl[unit])
        n261 = local read "Ch2Duty (%) Set"() -> (w388:dbl)
        n262 = local read "OverallPeriodSet"() -> (w385:dbl[unit])
        n263 = local read "Width/Duty\nUP/DOWN Ch2"() -> (w383:bool)
        n264 = Divide(x=w388, y=100.0) -> (x/y=w386:dbl)
        n265 = Multiply(x=w386, y=w385) -> (x*y=w384:dbl[unit])
        n266 = Select(t=w382, s=w383, f=w384) -> (s? t:f=w381:dbl[unit])
        n267 = local write "Ch2WidthSet"(w381) -> ()
      }
      event #16 {
        n268 = event-data() -> ("NewVal"=w395:dbl[unit])  [unwired: 6 out]
        n269 = local read "OverallPeriodSet"() -> (w394:dbl[unit])
        n270 = Divide(x=w395, y=w394) -> (x/y=w393:dbl)
        n271 = Multiply(x=100, y=w393) -> (x*y=w391:dbl)
        n272 = local write "Ch1Duty (%) Set"(w391) -> ()
      }
      event #17 {
        n273 = event-data() -> ("NewVal"=w398:dbl[unit])  [unwired: 6 out]
        n274 = local read "OverallPeriodSet"() -> (w402:dbl[unit])
        n275 = Divide(x=w398, y=w402) -> (x/y=w401:dbl)
        n276 = Multiply(x=100, y=w401) -> (x*y=w399:dbl)
        n277 = local write "Ch2Duty (%) Set"(w399) -> ()
      }
    }
    n278 = call-dynamic "VISA Get Session.vi"("error in (no error)"=w22, "Instrument.lvclass in"=w23) -> ("error out"=w21:errorcluster, "VISA Resource Name"=w27:refnum<visa-resource-name>, "Instrument.lvclass out"=w25:refnum<class "Pulse Generator.lvclass">)  [unwired: 7 out]
    n279 = call "HP81110A Error Query.vi"("VISA session"=w27, "error in (no error)"=w21) -> ("dup VISA session"=w26:refnum<visa-resource-name>, "error out"=w30:errorcluster)  [unwired: 12 out]
    n280 = call <vilib>:"Simple Error Handler.vi"("error in (no error)"=w30) -> ("error out"=w20:errorcluster)  [unwired: 1 in, 7 out]
    n281 = call-dynamic "VISA Save Session.vi"("error in (no error)"=w20, "VISA Resource Name"=w26, "Instrument.lvclass in"=w25) -> ("error out"=w19:errorcluster, "Instrument.lvclass out"=w24:refnum<class "Pulse Generator.lvclass">)  [unwired: 7 out]
  }
  n282 = call-dynamic "_Destroy.vi"("error in (no error)"=w12, "Instrument in"=w13) -> ("error out"=→"error out":errorcluster)  [unwired: 9 out]
